vi "LED (SubVI).vi"(2 "error in (no error)":errorcluster, 3 "LINX Resource in":T1, 4 "Blue / Red":bool, 5 "On/OFF":bool) -> (0 "error out":errorcluster, 1 "LINX Resource out":T1)   [LabVIEW 2020]
uses:
  <vilib>/MakerHub/LINX/Private/Type Defs/LINX Ref.ctl
  <vilib>/MakerHub/LINX/Private/Type Defs/Platform.ctl
  <vilib>/MakerHub/LINX/Private/Type Defs/Interface.ctl
  <vilib>/MakerHub/LINX/Private/Device/Type Defs/LINX Device Config.ctl
  <vilib>/MakerHub/LINX/Private/Device/Type Defs/TCP Config.ctl
  <vilib>/MakerHub/LINX/Private/Device/Type Defs/Channels.ctl
  <vilib>/MakerHub/LINX/Public/Peripherals/Digital/Digital Write N Chans.vi
  <vilib>/MakerHub/LINX/Private/Local IO/LinxDigitalWrite.vi
  <vilib>/MakerHub/LINX/Public/Utilities/Check Channel.vi
  <vilib>/MakerHub/LINX/Private/Utilties/Generate Error.vi
  <vilib>/MakerHub/LINX/LMH-LINX.lvlib
  <vilib>/MakerHub/LINX/Private/Device/Device.lvlib
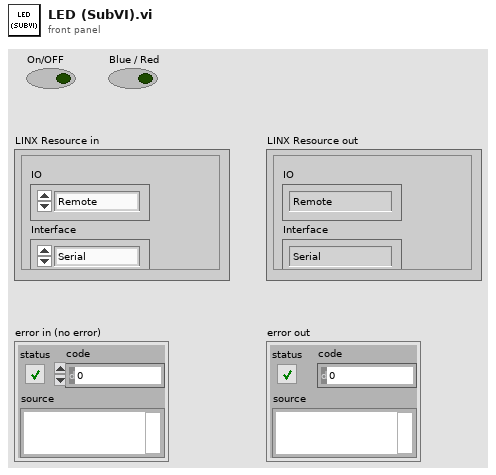
[diagram p1: front panel]
types:
  T1 = typedef "LMH-LINX.lvlib/LINX Ref.ctl" = cluster{"IO":T2, "Interface":T3, "LINX Device Config":T4}
  T2 = typedef "LMH-LINX.lvlib/Platform.ctl" = enum16{"Remote", "Local"}
  T3 = typedef "LMH-LINX.lvlib/Interface.ctl" = enum16{"Serial", "TCP"}
  T4 = typedef "LMH-LINX.lvlib/Device.lvlib/LINX Device Config.ctl" = cluster{"Interface":T3, "COM Port":refnum<visa-resource-name>, "TCP Configuration":T5, "Device Family":u8, "Device ID":u8, "Device Name":string, "TCP Ref":refnum<k5>, "Channels":T6}
  T5 = typedef "LMH-LINX.lvlib/Device.lvlib/TCP Config.ctl" = cluster{"IP Address":string, "Port":u16}
  T6 = typedef "LMH-LINX.lvlib/Channels.ctl" = cluster{"DI":u8[], "DO":u8[], "AI":u8[], "AO":u8[], "PWM":u8[], "QE":u8[], "UART":u8[], "I2C 2":u8[], "SPI":u8[], "CAN":u8[], "Servo":u8[], "AI Ref (V)":dbl, "AI Resolution (Bits)":u8, "AO Ref (V)":dbl, "AO Resolution (Bits)":u8}
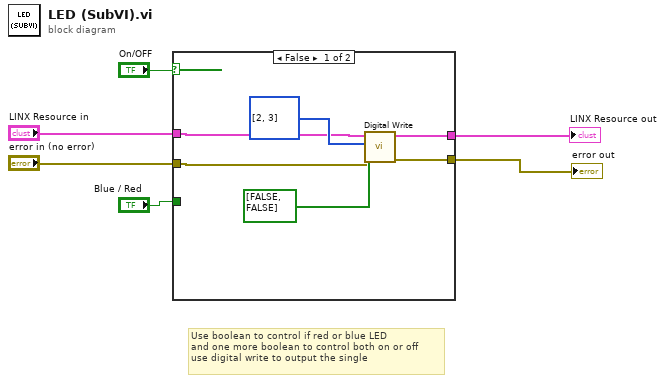
[diagram p0: block diagram]
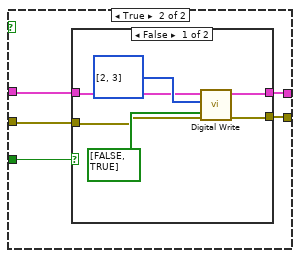
[diagram p2: hidden frame]
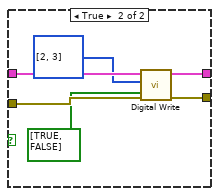
[diagram p3: hidden frame]
diagram:
  # "Use boolean to control if red or blue LED \nand one more boolean to control both on or off\nuse digital write to output the single"
  n1 = case shown="False" "On/OFF" {
    tunnel: "error in (no error)" -> [w9 w17]
    tunnel: "LINX Resource in" -> [w10 w16]
    tunnel: [w8 w15] -> w4
    tunnel: [w7 w14] -> w5
    tunnel: "Blue / Red" -> [_ w13]
    frame False {
      n2 = call-poly <vilib>:"Digital Write.vi"("Error In"=w9, "Values"=bool[] [FALSE, FALSE], "DO Channels"=u8[] [2, 3], "LINX Resource"=w10) -> ("Error Out"=w7:errorcluster, "LINX Resource"=w8:T1)  [unwired: 6 in]
    }
    frame True {
      n3 = case shown="False" w13 {
        tunnel: w17 -> [w20 w29]
        tunnel: w16 -> [w21 w28]
        tunnel: [w19 w25] -> w15
        tunnel: [w18 w24] -> w14
        frame False {
          n4 = call-poly <vilib>:"Digital Write.vi"("Error In"=w20, "Values"=bool[] [FALSE, TRUE], "DO Channels"=u8[] [2, 3], "LINX Resource"=w21) -> ("Error Out"=w18:errorcluster, "LINX Resource"=w19:T1)  [unwired: 6 in]
        }
        frame True {
          n5 = call-poly <vilib>:"Digital Write.vi"("Error In"=w29, "Values"=bool[] [TRUE, FALSE], "DO Channels"=u8[] [2, 3], "LINX Resource"=w28) -> ("Error Out"=w24:errorcluster, "LINX Resource"=w25:T1)  [unwired: 6 in]
        }
      }
    }
  }
  "error out" <- w5
  "LINX Resource out" <- w4
